vi "Simple Connection Settings Polymorphic.vi"(6 "Simple Connection Settings":T1, 8 "error in (no error)":errorcluster, 10 "XML Elements":string) -> (0 "error out":errorcluster, 1 "VISA resource name":T1)   [LabVIEW 2014]
uses:
  Controls/Simple Connection Settings Cluster.ctl
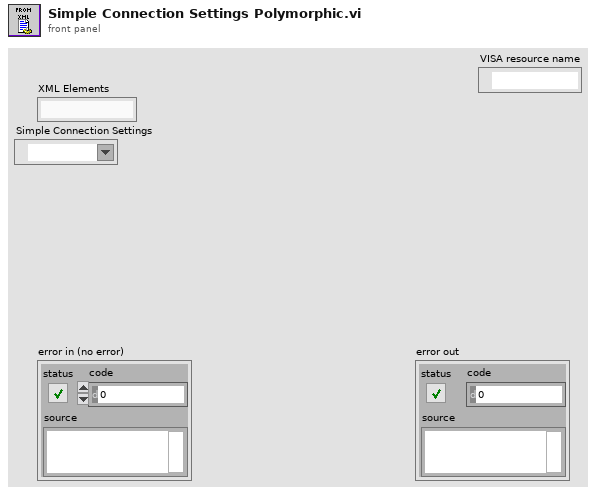
[diagram p1: front panel]
types:
  T1 = typedef "Simple Connection Settings Cluster.ctl" = refnum<visa-resource-name>
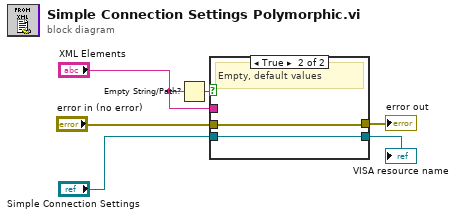
[diagram p0: block diagram]
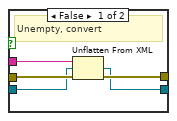
[diagram p2: hidden frame]
diagram:
  n1 = Empty String/Path?(string/path="XML Elements") -> (empty?=w3:bool)
  n2 = case shown="True" w3 {
    tunnel: "error in (no error)" -> [w11 w12]
    tunnel: "Simple Connection Settings" -> [w8 w13]
    tunnel: [w7 w13] -> w1
    tunnel: [w10 w12] -> w5
    tunnel: "XML Elements" -> [w9 _]
    frame False {
      # "Unempty, convert"
      n3 = Unflatten From XML(xml string=w9, type=w8, error in (no error)=w11) -> (value=w7:T1, error out=w10:errorcluster)
    }
    frame True {
      # "Empty, default values"
    }
  }
  "error out" <- w5
  "VISA resource name" <- w1
